vi "2_Objects_Detection(Eval).vi"() -> ()   [LabVIEW 2020]
uses:
  <vilib>/Ngene/Deep Learning Toolkit/Toolkit/NN_Network/Controls/NN_Device.ctl
  <vilib>/Ngene/Deep Learning Toolkit/Toolkit/NN_Network/Controls/NN_Save_Before_Destroy_Options.ctl
  <vilib>/Ngene/Deep Learning Toolkit/Toolkit/NN_Network/subVIs/NN_Predict/NN_Predict(In3D_OutBBox).vi
  <vilib>/Ngene/Deep Learning Toolkit/Toolkit/NN_Train/Eval_Loss/NN_Eval_Test_Error_Loss/NN_Eval(In3D_OutBBox).vi
  <vilib>/Ngene/Deep Learning Toolkit/Toolkit/NN_Train/Eval_Loss/NN_Calc_Cofusion_Matrix/NN_Calc_Confusion_Matrix(In3D_OutBBox).vi
  <vilib>/Ngene/Deep Learning Toolkit/Toolkit/Deep_Learning_Toolkit_by_Ngene.lvlib
panel:
  out "Confusion Matrix":string[][](table)=[["455", "0", "0", "1", "0.9978"], ["0", "398", "0", "5", "0.9876"], ["0", "0", "373", "3", "0.9920"], ["1", "11", "0", "0", "0.0000"], ["0.9978", "0.9731", "1.0000", "0.0000", ""]]
  out "mIOU":sgl=0.8852882 format="%#_3g"
  out "mAP@0.5":sgl=0.9981299 format="%#_3g"
  out "APs@0.5 Per Class":sgl[](array[numeric])=[0.9999759, 0.9945516, 0.9998622] format="%#_3g"
  out "Optml Conf Thresh":sgl=0.278 format="%#_3g"
  out "Labels":string[](array[string])=["Nut", "Screw", "Washer"]
  out "Dataset_Size":i32=74
  out "IOUs Per Class":sgl[](array[numeric])=[0.8858802, 0.8480403, 0.9219441] format="%#_3g"
  in  "mBatch":i32=32
  out "Precision":sgl=0.99030405 format="%#_3g"
  out "Recall":sgl=0.9933603 format="%#_3g"
  out "Avg_F1,P,R Curves":cluster{"Conf":sgl[], "F1|P|R":sgl[]}[](graph)
  in  "Dataset (Annotations)":path=path "D:/Ngene/GitHub/deepltk_examples/3_Image_Processing/33_Object_Detection/Dataset/Orig/Test/Annotations"
  in  "Dataset (Images)":path=path "D:/Ngene/GitHub/deepltk_examples/3_Image_Processing/33_Object_Detection/Dataset/Orig/Test/Images"
  in  "NMS_IOU_Thrsh":sgl=0.45 format="%#_3g"
  in  "NN_Device":T1=enum."GPU"
  in  "Model Weights":path=path "D:/Ngene/GitHub/deepltk_examples/3_Image_Processing/33_Object_Detection/Trained Model/512x910_mAP_0.998/Obj_Det_Example_weights_25_06_09__13_45_53.bin"
  in  "Model Topology":path=path "D:/Ngene/GitHub/deepltk_examples/3_Image_Processing/33_Object_Detection/Trained Model/512x910_mAP_0.998/Obj_Det_Example_net_cfg_25_06_09__13_45_53.cfg"
  # "Overview:\nThis VI demonstrates how to evaluate performance of a trained model for a object detections.\nRequirements: Deep Learning Toolkit for LabVIEW.\nInstructions:\n1. Provide network topology .cfg file in the \"Model Topology\" control and trained weights .bin file in the \"Model Weights\" control.\n2. Provide path to the folder with test images and annotations at \"Dataset (Images)\" and \"Dataset (Annotations)\" \n3. Run the VI to evaluate the model's performance."
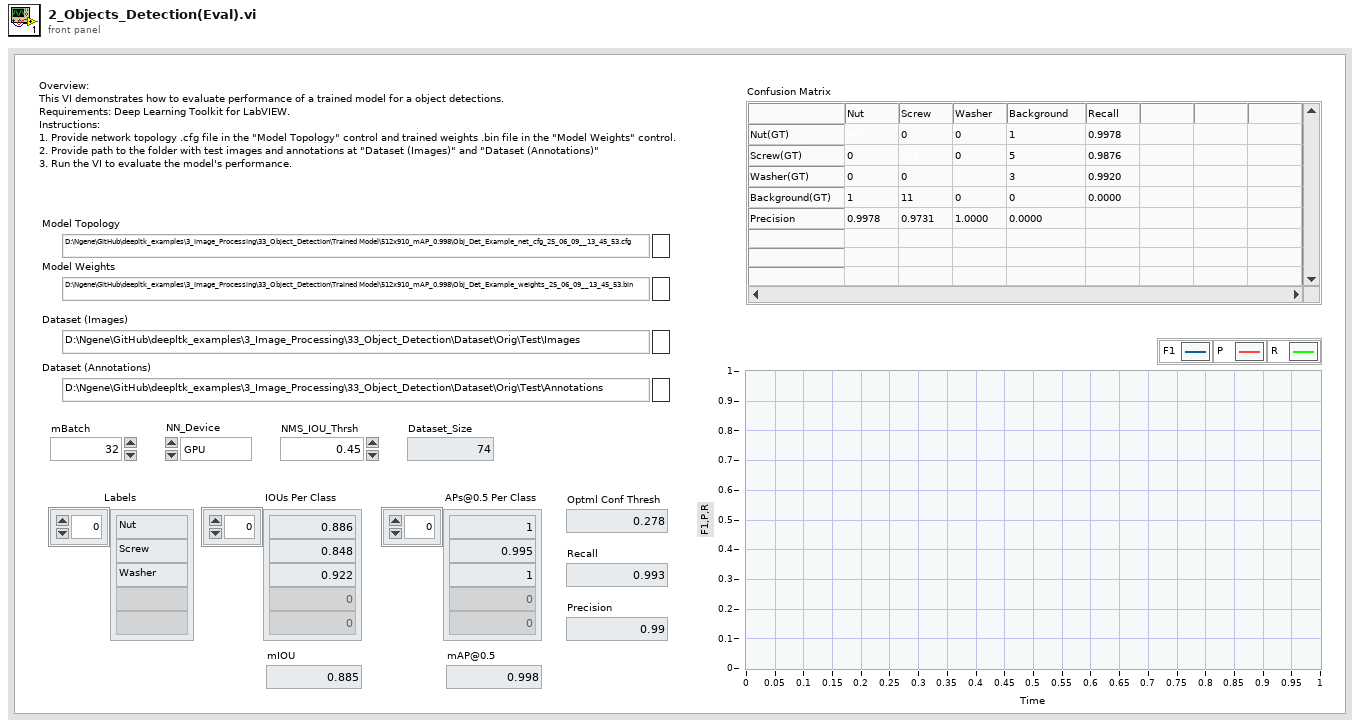
[diagram p1: front panel]
types:
  T1 = typedef "Deep_Learning_Toolkit_by_Ngene.lvlib/NN_Device.ctl" = enum16{"CPU", "GPU"}
  T2 = typedef "Deep_Learning_Toolkit_by_Ngene.lvlib/NN_Save_Before_Destroy_Options.ctl" = cluster{"CFG?":bool, "Weights?":bool, "Render?":bool}
  T3 = typedef "Deep_Learning_Toolkit_by_Ngene.lvlib/NN_Config_Params.ctl" = cluster{"Name":string, "mBatch":i32, "NN_Train_Params":T4, "LR_Decay_Policy":T7, "Labels":string[], "Loss":T9}
  T4 = typedef "Deep_Learning_Toolkit_by_Ngene.lvlib/NN_Train_Params.ctl" = cluster{"Optimizer":T5, "Beta_1":sgl, "Beta_2":sgl, "Weight Decay(L1)":sgl, "Weight Decay(L2)":sgl, "Data_Sampling":T6}
  T5 = typedef "Deep_Learning_Toolkit_by_Ngene.lvlib/NN_Train_Optimizer.ctl" = enum16{"SGD", "Adam", "Adagrad", "Adadelta", "RMSProp", "Nesterov"}
  T6 = typedef "Deep_Learning_Toolkit_by_Ngene.lvlib/NN_Train_Data_Sampling.ctl" = enum16{"Random", "Sequential"}
  T7 = typedef "Deep_Learning_Toolkit_by_Ngene.lvlib/NN_LR_Policy_Cfg.ctl" = cluster{"Policy_Type":T8, "LR0":dbl, "k":sgl, "WarmUp_Policy":enum16{"Step", "Ramp"}, "WarmUp_Iter":i32, "WarmUp_Ratio":sgl}
  T8 = typedef "Deep_Learning_Toolkit_by_Ngene.lvlib/NN_LR_Policy_Type.ctl" = enum16{"Manual", "Step", "Exp", "1/t"}
  T9 = typedef "Deep_Learning_Toolkit_by_Ngene.lvlib/NN_Loss_Config_Params.ctl" = cluster{"Loss_Type":T10, "Loss_Conf_Params":variant}
  T10 = typedef "Deep_Learning_Toolkit_by_Ngene.lvlib/NN_Loss_Type.ctl" = enum16{"None", "MSE", "CrossEntropy", "YOLO_v2", "YOLO_v4"}
  T11 = typedef "Deep_Learning_Toolkit_by_Ngene.lvlib/NN_Layer_Config_Params.ctl" = cluster{"Layer_Type":T12, "Layer_Conf_Params":variant, "Input Layers":string[]}
  T12 = typedef "Deep_Learning_Toolkit_by_Ngene.lvlib/NN_Layer_Type.ctl" = enum16{"Input1D", "Input3D", "Conv1D", "Conv2D", "Conv2D_Adv", "MaxPool", "AvgPool", "UpSample", "DropOut3D", "ShortCut", "Concat", "SoftMax3D", "FC", "DropOut", "Softmax", "Flatten", "YOLO_v2", "YOLO_v4", "Activation", "BatchNormalization", "Unsupported"}
  T13 = typedef "Deep_Learning_Toolkit_by_Ngene.lvlib/NN.ctl" = cluster{"Name":string, "No of Layers":i32, "mBatch":i32, "Layers":T14[], "Dimty":T15, "Dims_In":T16, "Dims_Out":T16, "Working_Dir":path, "Train?":bool, "Train_Params":T4, "LR_Update_Policy":T7, "Session Data":T17, "Ground_truth":T18, "NNg_hdls":T19, "NN_Device":T1, "GPU Id":i32, "Labels":string[], "Receptive Field":T20[], "Loss_Type":T10, "Loss_Cfg_Prms":variant, "NNG_WS":T21}
  T14 = typedef "Deep_Learning_Toolkit_by_Ngene.lvlib/NN_Layer_ref.ctl" = refnum<data-value>
  T15 = typedef "Deep_Learning_Toolkit_by_Ngene.lvlib/NN_In_Out_Dim-ty.ctl" = enum8{"In1D_Out1D", "In3D_Out1D", "In3D_Out3D", "In3D_OutBBox"}
  T16 = typedef "Deep_Learning_Toolkit_by_Ngene.lvlib/NN_Dims(C,H,W).ctl" = cluster{"C":i32, "H":i32, "W":i32}
  T17 = typedef "Deep_Learning_Toolkit_by_Ngene.lvlib/NN_Train_Session_Data.ctl" = cluster{"Epochs":sgl, "Tot_Iter":i32, "LR":sgl, "LR_iter":i32}
  T18 = typedef "Deep_Learning_Toolkit_by_Ngene.lvlib/NN_Ground_truth.ctl" = cluster{"Y":variant}
  T19 = typedef "Deep_Learning_Toolkit_by_Ngene.lvlib/nng_cuda_handles.ctl" = cluster{"cudnn":u64, "cublas":u64, "stream":u64, "curand":u64}
  T20 = typedef "Deep_Learning_Toolkit_by_Ngene.lvlib/NN_Dims(V,H).ctl" = cluster{"V":i32, "H":i32}
  T21 = typedef "Deep_Learning_Toolkit_by_Ngene.lvlib/NNG_WS.ctl" = cluster{"NNG_WS_Mem":T22, "Max_WS_Size":i64}
  T22 = typedef "Deep_Learning_Toolkit_by_Ngene.lvlib/NNg_WS_Mem_DVR.ctl" = refnum<data-value>
  T23 = typedef "Deep_Learning_Toolkit_by_Ngene.lvlib/NN_DataSet(In3D_OutBBox).ctl" = cluster{"Inputs Ref.":variant, "Dataset_Size":i32, "Dims_In":T16, "Outputs Refs":T24, "No of Classes ":i32, "Labels":string[], "File Paths":path[]}
  T24 = typedef "Deep_Learning_Toolkit_by_Ngene.lvlib/NN_Data_ref(1D_BBox).ctl" = refnum<data-value>
  T25 = typedef "Deep_Learning_Toolkit_by_Ngene.lvlib/NN_Image_Detections.ctl" = cluster{"Image Detections":T26[]}
  T26 = typedef "Deep_Learning_Toolkit_by_Ngene.lvlib/NN_BBox_Detection.ctl" = cluster{"Class":i32, "Conf Level":sgl, "BBox":T27}
  T27 = typedef "Deep_Learning_Toolkit_by_Ngene.lvlib/NN_BBox.ctl" = cluster{"x":sgl, "y":sgl, "w":sgl, "h":sgl}
  T28 = typedef "Deep_Learning_Toolkit_by_Ngene.lvlib/NN_Eval_Params(in3D_OutBBox).ctl" = cluster{"Precision@Max_Avg_F1_Score":sgl, "Recall@Max_Avg_F1_Score":sgl, "argmax_avgF1_Score(Conf)":sgl, "Max_Avg_F1_Score":sgl, "Max_F1_Score_Per_Class":sgl[], "F1_Score_Per_Class":sgl[][], "Avg_F1,P,R Curves":cluster{"Conf":sgl[], "F1|P|R":sgl[]}[], "mIOU":sgl, "APs@0.5":sgl[], "PR_Curves@0.5":T29, "IOUs":sgl[], "mAP@0.75":sgl, "mAP@0.5-0.95":sgl, "mAP@0.5":sgl, "Mean_PR_Curve":T30}
  T29 = typedef "Deep_Learning_Toolkit_by_Ngene.lvlib/NN_PR_Curves.ctl" = T30[]
  T30 = typedef "Deep_Learning_Toolkit_by_Ngene.lvlib/NN_PR.ctl" = cluster{"Recall":sgl[], "Precision":sgl[]}
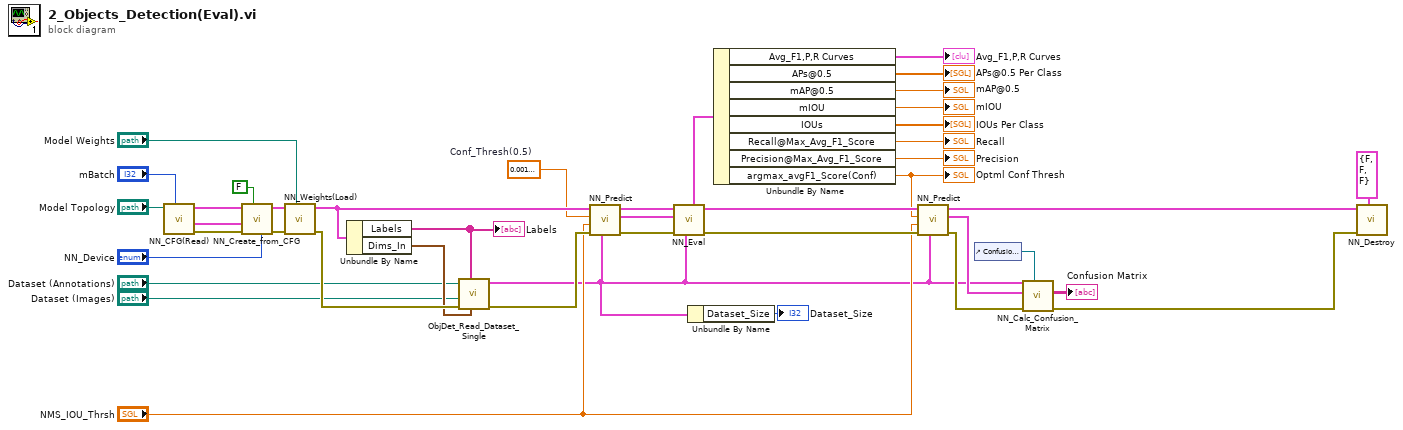
[diagram p0: block diagram]
diagram:
  w28 = sgl 0.001  # Conf_Thresh(0.5)
  n1 = call <vilib>:"NN_CFG(Read).vi"("mBatch"="mBatch", "CFG file path"="Model Topology") -> ("error out"=w40:errorcluster, "Net_Cfg"=w36:T3, "Layer_Cfg"=w41:T11[])  [unwired: 7 in]
  n2 = call <vilib>:"NN_Create_from_CFG.vi"("NN_Device"="NN_Device", "Train? (false)"=FALSE, "error in (no error)"=w40, "Net_Cfg"=w36, "Layer_Cfg"=w41) -> ("error out"=w39:errorcluster, "NN out"=w37:T13)  [unwired: 5 in]
  n3 = call <vilib>:"NN_Weights(Load).vi"("Weight File Path"="Model Weights", "error in (no error)"=w39, "NN in"=w37) -> ("error out"=w32:errorcluster, "NN out"=w31:T13)  [unwired: 7 in]
  n4 = Unbundle By Name(w31) -> ("Labels"=w1:string[], "Dims_In"=w23:T16)
  "Labels" <- w1
  n5 = call "ObjDet_Read_Dataset_Single.vi"("Dims(C,H,W)"=w23, "Unique labels"=w1, "error in (no error)"=w32, "Dataset Path (Images)"="Dataset (Images)", "Annotations Path"="Dataset (Annotations)") -> ("error out"=w30:errorcluster, "NN_DataSet(In3D_OutBBox)"=w4:T23)  [unwired: 4 in, 1 out]
  n6 = call-poly <vilib>:"NN_Predict.vi"("Dataset"=w4, "error in (no error)"=w30, "NMS_IOU_Thresh(0.5)"="NMS_IOU_Thrsh", "Conf_Thresh(0.5)"=w28, "NN in"=w31) -> ("error out"=w26:errorcluster, "Predictions"=w22:T25[], "NN out"=w25:T13)  [unwired: 4 in]
  n7 = call-poly <vilib>:"NN_Eval.vi"("Dataset"=w4, "error in"=w26, "Detections(in Dataset)"=w22, "NN in"=w25) -> ("error out"=w11:errorcluster, "NN out"=w13:T13, "NN_Eval_Params"=w24:T28)  [unwired: 5 in]
  n8 = Unbundle By Name(w4) -> ("Dataset_Size"=→"Dataset_Size":i32)
  n9 = Unbundle By Name(w24) -> ("Avg_F1,P,R Curves"=→"Avg_F1,P,R Curves":cluster{"Conf":sgl[], "F1|P|R":sgl[]}[], "APs@0.5"=→"APs@0.5 Per Class":sgl[], "mAP@0.5"=→"mAP@0.5":sgl, "mIOU"=→"mIOU":sgl, "IOUs"=→"IOUs Per Class":sgl[], "Recall@Max_Avg_F1_Score"=→"Recall":sgl, "Precision@Max_Avg_F1_Score"=→"Precision":sgl, "argmax_avgF1_Score(Conf)"=w9:sgl)
  "Optml Conf Thresh" <- w9
  n10 = call-poly <vilib>:"NN_Predict.vi"("Dataset"=w4, "error in (no error)"=w11, "NMS_IOU_Thresh(0.5)"="NMS_IOU_Thrsh", "Conf_Thresh(0.5)"=w9, "NN in"=w13) -> ("error out"=w10:errorcluster, "Predictions"=w7:T25[], "NN out"=w12:T13)  [unwired: 4 in]
  n11 = control-ref of="Confusion Matrix"() -> (w6:refnum<vi>)
  n12 = call-poly <vilib>:"NN_Calc_Confusion_Matrix.vi"("Confusion Matrix (Table) ref."=w6, "error in (no error)"=w10, "Predictions"=w7, "Dataset"=w4) -> ("error out"=w15:errorcluster, "Confusion Matrix (Table)"=→"Confusion Matrix":string[][])  [unwired: 4 in, 2 out]
  n13 = call <vilib>:"NN_Destroy.vi"("Save (T, T, T)"=T2 {"CFG?"=FALSE, "Weights?"=FALSE, "Render?"=FALSE}, "error in (no error)"=w15, "NN in"=w12) -> ()  [unwired: 7 in, 2 out]
